vi "BRig_FPGA_sinwave_build.vi"(11 "input_Npts":i32=100) -> (3 "output_array_sin":fxp<+/-,16,2>[](array[numeric]))   [LabVIEW 2014]
uses:
  <vilib>/rvi/FXPMathLib/FxpDiv/subVIs/nifxpmath_Div_SimConfig.ctl
  <vilib>/rvi/FXPMathLib/FxpSinAndCos/subVIs/nifxpmath_SinAndCos_SimConfig.ctl
  <vilib>/rvi/FXPMathLib/FxpDiv/simVIs/DllFxpDivTemp_sub.vi
  <vilib>/rvi/FXPMathLib/FxpSinAndCos/simVIs/DllFxpSinAndCosTemp_sub.vi
  <vilib>/rvi/FXPMathLib/FxpDiv/XNode/nifxpmath_Div.xnode
  <vilib>/rvi/FXPMathLib/FxpMul/XNode/nifxpmath_Multiplier.xnode
  <vilib>/rvi/FXPMathLib/FxpSinAndCos/XNode/nifxpmath_SinAndCos.xnode
  <vilib>/rvi/FXPMathLib/sim/FxpSim.dll
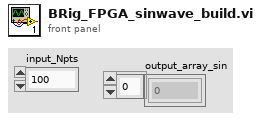
[diagram p1: front panel]
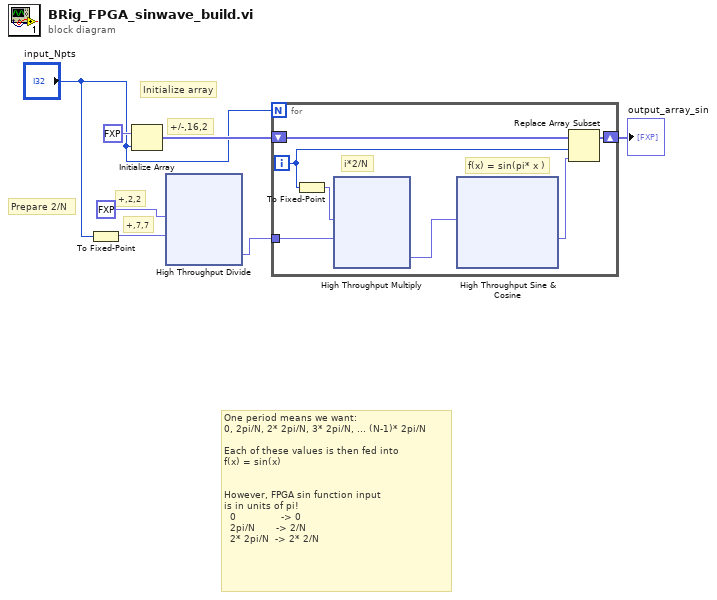
[diagram p0: block diagram]
diagram:
  # "+,7,7"
  # "+,2,2"
  # "+/-,16,2"
  # "Prepare 2/N"
  # "One period means we want:\n0, 2pi/N, 2* 2pi/N, 3* 2pi/N, ... (N-1)* 2pi/N\n\nEach of these values is then fed into\nf(x) = sin(x)\n\n\nHowever, FPGA sin function input\nis in units of pi!\n  0               -> 0\n  2pi/N       -> 2/N\n  2* 2pi/N  -> 2* 2/N"
  # "Initialize array"
  n1 = To Fixed-Point(number="input_Npts") -> (fixed-point=w4:fxp<+,7,7>)  [unwired: 1 in]
  n2 = Initialize Array(fxp<+/-,16,2> 0.0 ("element"), "input_Npts") -> (w7:fxp<+/-,16,2>[])
  n3 = xnode "High Throughput Divide"("x"=fxp<+,2,2> 2.0, "y"=w4) -> ("x/y"=w3:fxp<+,27,0>)
  n4 = for {
    N: "input_Npts" -> [_]
    shift-right: [w13] -> w1
    shift-left: w7 -> [w14]
    tunnel: w3 -> [w9]
    i -> [w12]
    # "f(x) = sin(pi* x )"
    # "i*2/N"
    n5 = To Fixed-Point(number=w12) -> (fixed-point=w10:fxp<+,7,7>)  [unwired: 1 in]
    n6 = xnode ("High Throughput Multiply")("x"=w10, "y"=w9) -> ("x*y"=w8:fxp<+,34,7>)
    n7 = xnode "High Throughput Sine & Cosine"("x (pi)"=w8) -> ("sin(x)"=w11:fxp<+/-,16,2>)  [unwired: 1 out]
    n8 = Replace Array Subset(array=w14, new element=w11, index=w12) -> (w13:fxp<+/-,16,2>[])
  }
  "output_array_sin" <- w1
